vi "Add.vi"(1 "y":i32, 2 "x":i32) -> (0 "x+y":i32)   [LabVIEW 2016]
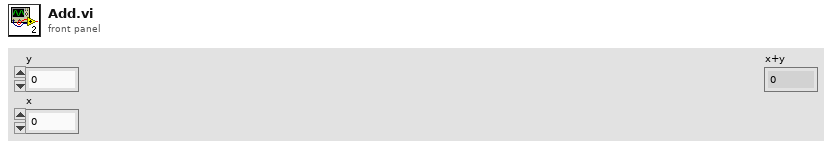
[diagram p1: front panel]
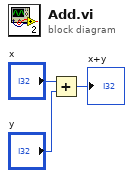
[diagram p0: block diagram]
diagram:
  n1 = Add(x="x", y="y") -> (x+y=→"x+y":i32)
